vi "Shared Memory Example.vi"() -> ()   [LabVIEW 2017]
uses:
  lib/sm bool read and increment.vi
  lib/sm double read and increment.vi
  lib/sm single read and increment.vi
  lib/sm i64 read and increment.vi
  lib/sm i32 read and increment.vi
  lib/sm i16 read and increment.vi
  lib/sm i8 read and increment.vi
  lib/sm u64 read and increment.vi
  lib/sm u32 read and increment.vi
  lib/sm u16 read and increment.vi
  lib/sm u8 read and increment.vi
  lib/sm double write and increment.vi
  lib/sm single write and increment.vi
  lib/sm i64 write and increment.vi
  lib/sm i32 write and increment.vi
  lib/sm i16 write and increment.vi
  lib/sm i8 write and increment.vi
  lib/sm u64 write and increment.vi
  lib/sm u32 write and increment.vi
  lib/sm u16 write and increment.vi
  lib/sm u8 write and increment.vi
  lib/sm bool write and increment.vi
  lib/linuxSharedMemory.lvlib
panel:
  in  "Boolean in":bool
  in  "U8":u8
  in  "U16":u16
  in  "U32":u32
  in  "U64":u64
  in  "I8":i8
  in  "I16":i16
  in  "I32":i32
  in  "I64":i64
  in  "Single":sgl
  in  "double":dbl
  out "U8":u8
  out "U16":u16
  out "U32":u32
  out "U64":u64
  out "I8":i8
  out "I16":i16
  out "I32":i32
  out "I64":i64
  out "Single":sgl
  out "double":dbl
  out "Boolean":bool
  in  "stop":bool
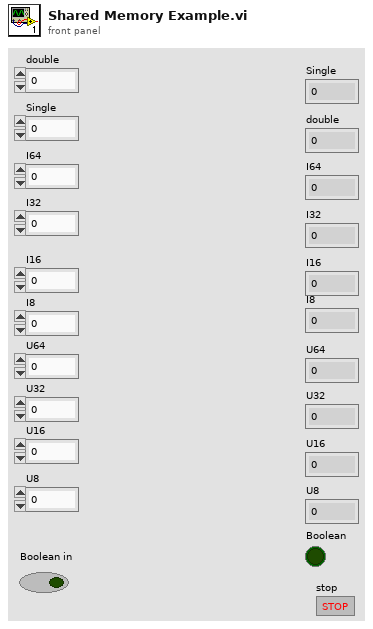
[diagram p1: front panel]
types:
  T1 = typedef "Linux RT IPC.Shared Memory.lvlib/reference.ctl" = refnum<data-value>
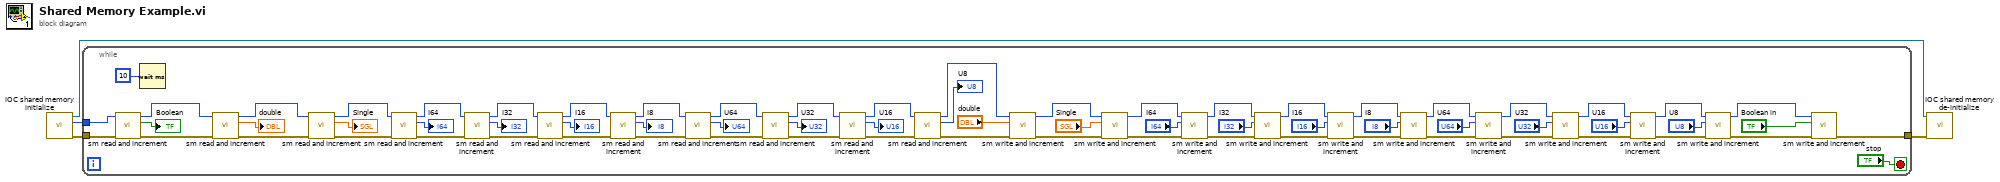
[diagram p0: block diagram]
diagram:
  n1 = call "IOC shared memory initialize.vi"() -> ("error out"=w3:errorcluster, "pointer to shared memory"=w2:u64, "shared memory out"=w4:T1)  [unwired: 9 in]
  n2 = while {
    tunnel: w3 -> [w71]
    tunnel: w2 -> [w72]
    tunnel: [w38] -> w1
    stop <- "stop" stop-if-true
    n3 = call-poly "sm read and increment.vi"("error in (no error)"=w71, "pointer in"=w72) -> ("error out"=w69:errorcluster, "Bool out"=→"Boolean":bool, "Shared Memory PTR out"=w61:u64)  [unwired: 7 in]
    n4 = Wait (ms)(milliseconds to wait=10) -> ()  [unwired: 1 out]
    n5 = call-poly "sm read and increment.vi"("error in (no error)"=w69, "pointer in"=w61) -> ("error out"=w68:errorcluster, "value out"=→"double":dbl, "Shared Memory PTR out"=w60:u64)  [unwired: 7 in]
    n6 = call-poly "sm read and increment.vi"("error in (no error)"=w68, "pointer in"=w60) -> ("error out"=w67:errorcluster, "value out"=→"Single":sgl, "Shared Memory PTR out"=w59:u64)  [unwired: 7 in]
    n7 = call-poly "sm read and increment.vi"("error in (no error)"=w67, "pointer in"=w59) -> ("error out"=w66:errorcluster, "value out"=→"I64":i64, "Shared Memory PTR out"=w58:u64)  [unwired: 7 in]
    n8 = call-poly "sm read and increment.vi"("error in (no error)"=w66, "pointer in"=w58) -> ("error out"=w65:errorcluster, "value out"=→"I32":i32, "Shared Memory PTR out"=w57:u64)  [unwired: 7 in]
    n9 = call-poly "sm read and increment.vi"("error in (no error)"=w65, "pointer in"=w57) -> ("error out"=w64:errorcluster, "value out"=→"I16":i16, "Shared Memory PTR out"=w56:u64)  [unwired: 7 in]
    n10 = call-poly "sm read and increment.vi"("error in (no error)"=w64, "pointer in"=w56) -> ("error out"=w63:errorcluster, "value out"=→"I8":i8, "Shared Memory PTR out"=w55:u64)  [unwired: 7 in]
    n11 = call-poly "sm read and increment.vi"("error in (no error)"=w63, "pointer in"=w55) -> ("error out"=w62:errorcluster, "value out"=→"U64":u64, "Shared Memory PTR out"=w54:u64)  [unwired: 7 in]
    n12 = call-poly "sm read and increment.vi"("error in (no error)"=w62, "pointer in"=w54) -> ("error out"=w53:errorcluster, "value out"=→"U32":u32, "Shared Memory PTR out"=w50:u64)  [unwired: 7 in]
    n13 = call-poly "sm read and increment.vi"("error in (no error)"=w53, "pointer in"=w50) -> ("error out"=w51:errorcluster, "value out"=→"U16":u16, "Shared Memory PTR out"=w52:u64)  [unwired: 7 in]
    n14 = call-poly "sm read and increment.vi"("error in (no error)"=w51, "pointer in"=w52) -> ("error out"=w27:errorcluster, "value out"=→"U8":u8, "Shared Memory PTR out"=w25:u64)  [unwired: 7 in]
    n15 = call-poly "sm write and increment.vi"("error in (no error)"=w27, "value in"="double", "pointer in"=w25) -> ("error out"=w28:errorcluster, "Shared Memory PTR out"=w24:u64)  [unwired: 7 in]
    n16 = call-poly "sm write and increment.vi"("error in (no error)"=w28, "value in"="Single", "pointer in"=w24) -> ("error out"=w29:errorcluster, "Shared Memory PTR out"=w23:u64)  [unwired: 7 in]
    n17 = call-poly "sm write and increment.vi"("error in (no error)"=w29, "value in"="I64", "pointer in"=w23) -> ("error out"=w30:errorcluster, "Shared Memory PTR out"=w22:u64)  [unwired: 7 in]
    n18 = call-poly "sm write and increment.vi"("error in (no error)"=w30, "value in"="I32", "pointer in"=w22) -> ("error out"=w31:errorcluster, "Shared Memory PTR out"=w21:u64)  [unwired: 7 in]
    n19 = call-poly "sm write and increment.vi"("error in (no error)"=w31, "value in"="I16", "pointer in"=w21) -> ("error out"=w32:errorcluster, "Shared Memory PTR out"=w20:u64)  [unwired: 7 in]
    n20 = call-poly "sm write and increment.vi"("error in (no error)"=w32, "value in"="I8", "pointer in"=w20) -> ("error out"=w33:errorcluster, "Shared Memory PTR out"=w19:u64)  [unwired: 7 in]
    n21 = call-poly "sm write and increment.vi"("error in (no error)"=w33, "value in"="U64", "pointer in"=w19) -> ("error out"=w34:errorcluster, "Shared Memory PTR out"=w18:u64)  [unwired: 7 in]
    n22 = call-poly "sm write and increment.vi"("error in (no error)"=w34, "value in"="U32", "pointer in"=w18) -> ("error out"=w35:errorcluster, "Shared Memory PTR out"=w17:u64)  [unwired: 7 in]
    n23 = call-poly "sm write and increment.vi"("error in (no error)"=w35, "value in"="U16", "pointer in"=w17) -> ("error out"=w36:errorcluster, "Shared Memory PTR out"=w16:u64)  [unwired: 7 in]
    n24 = call-poly "sm write and increment.vi"("error in (no error)"=w36, "value in"="U8", "pointer in"=w16) -> ("error out"=w37:errorcluster, "Shared Memory PTR out"=w15:u64)  [unwired: 7 in]
    n25 = call-poly "sm write and increment.vi"("error in (no error)"=w37, "value in"="Boolean in", "pointer in"=w15) -> ("error out"=w38:errorcluster)  [unwired: 7 in, 1 out]
  }
  n26 = call "IOC shared memory de-initialize.vi"("shared memory in"=w4, "error in (no error)"=w1) -> ()  [unwired: 9 in]
